vi "write_login_info.vi"(7 "IP address":string, 8 "error in (no error)":errorcluster, 9 "Password":string, 10 "User":string, 11 "newport_xps in":refnum<class "newport_xps.lvclass">) -> (0 "error out":errorcluster, 3 "newport_xps out":refnum<class "newport_xps.lvclass">)   [LabVIEW 2015, in "newport_xps.lvclass"]
uses:
  newport_xps.lvclass
  newport_xps.lvclass/newport_xps.ctl
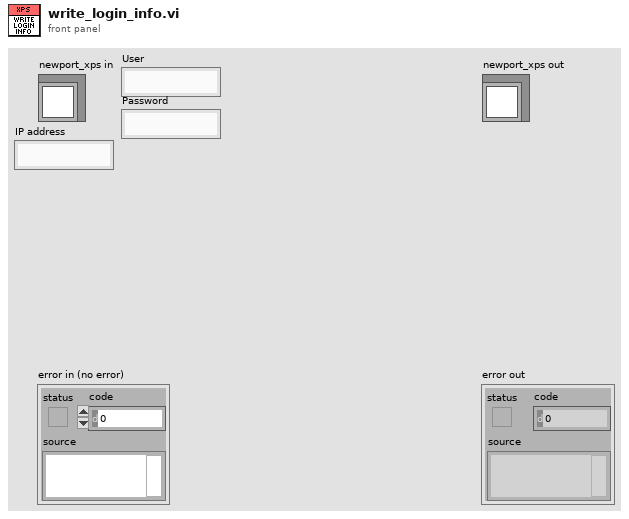
[diagram p1: front panel]
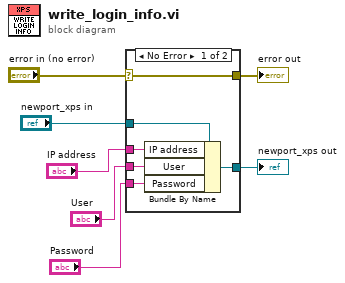
[diagram p0: block diagram]
diagram:
  n1 = case shown="No Error" "error in (no error)" {
    selector: "error in (no error)" -> [w13 w15]
    tunnel: [w13 w15] -> w6
    tunnel: [w10 w14] -> w4
    tunnel: "newport_xps in" -> [w12 w14]
    tunnel: "IP address" -> [w11 _]
    tunnel: "User" -> [w9 _]
    tunnel: "Password" -> [w8 _]
    frame No Error {
      n2 = Bundle By Name(cluster=w12, "IP address"=w11, "User"=w9, "Password"=w8) -> (w10:refnum<class "newport_xps.lvclass">)
    }
    frame Error {
    }
  }
  "error out" <- w6
  "newport_xps out" <- w4
